vi "UART Read Write.vi"() -> ()   [LabVIEW 2016]
panel:
  in  "Abort":bool
  in  "Start":bool
  out "error out":errorcluster
  in  "Send":bool
  in  "Command":string
  out "concatenated string":string
  in  "stop":bool
  in  "Boolean":bool
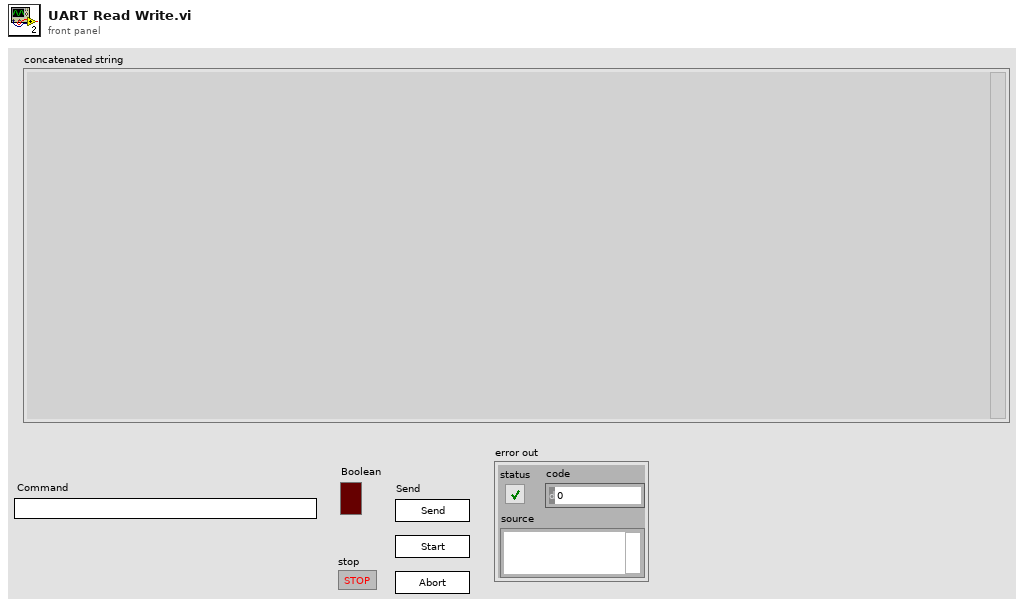
[diagram p1: front panel]
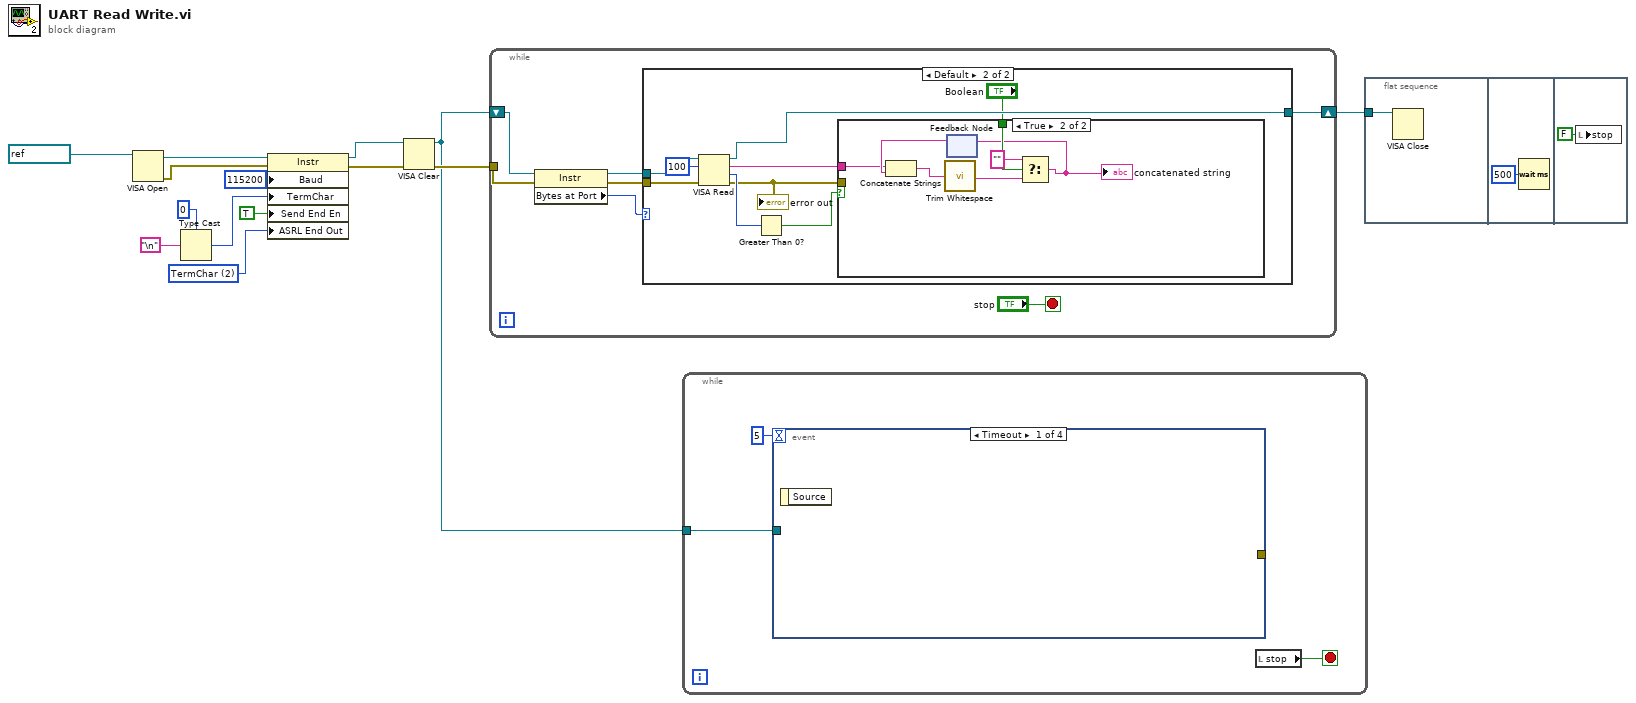
[diagram p0: block diagram]
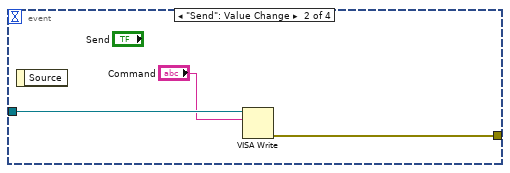
[diagram p2: hidden frame]
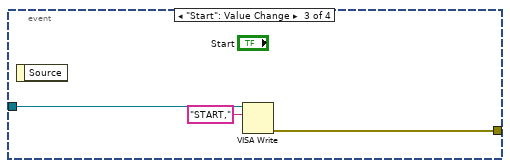
[diagram p3: hidden frame]
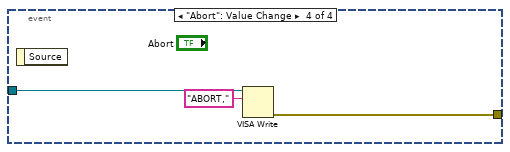
[diagram p4: hidden frame]
diagram:
  w4 = u16 2 items=["None", "Last Bit", "TermChar", "Break"] ("Serial Settings:End Mode for Writes")
  n1 = VISA Open(VISA resource name=refnum<visa-resource-name> "COM3") -> (VISA resource name=w13:refnum<visa-resource-name>, error out=w10:errorcluster)  [unwired: 4 in]
  n2 = Type Cast(type=u8 0 ("Message Based Settings:Termination Character"), x="\n") -> (*(type *) &x=w7:u8)
  n3 = property class="Instr"(reference=w13, error in=w10, "Baud"=u32 115200 ("Serial Settings:Baud Rate"), "TermChar"=w7, "Send End En"=TRUE ("Message Based Settings:Send End Enable"), "ASRL End Out"=w4) -> (reference out=w2:refnum<visa-resource-name>, error out=w11:errorcluster)
  n4 = VISA Clear(VISA resource name=w2, error in (no error)=w11) -> (VISA resource name out=w1:refnum<visa-resource-name>, error out=w3:errorcluster)
  n5 = while {
    tunnel: w3 -> [w17]
    shift-right: [w20] -> w9
    shift-left: w1 -> [w21]
    stop <- "stop" stop-if-true
    n6 = property class="Instr"(reference=w21, error in=w17) -> (reference out=w18:refnum<visa-resource-name>, error out=w16:errorcluster, "Bytes at Port"=w15:u32)
    n7 = case shown="Default" w15 {
      tunnel: [w22 w31] -> w20
      tunnel: w18 -> [w22 w24]
      tunnel: w16 -> [_ w23]
      frame 0 {
      }
      frame Default {
        n8 = VISA Read(VISA resource name=w24, byte count=u32 100, error in (no error)=w23) -> (VISA resource name out=w31:refnum<visa-resource-name>, read buffer=w30:string, return count=w26:u32, error out=w25:errorcluster)
        "error out" <- w25
        n9 = Greater Than 0?(x=w26) -> (x > 0?=w27:bool)
        n10 = case shown="True" w27 {
          tunnel: w30 -> [_ w36]
          tunnel: "Boolean" -> [_ w35]
          tunnel: w25 -> [_ _]
          frame False {
          }
          frame True {
            n11 = feedback #1() -> (w37:string)  [unwired: 1 in]
            n12 = Concatenate Strings(w36, w37) -> (w38:string)
            n13 = call <vilib>:"Trim Whitespace.vi"("string"=w38) -> ("trimmed string"=w34:string)  [unwired: 1 in]
            n14 = Select(t="", s=w35, f=w34) -> (s? t:f=w32:string)
            "concatenated string" <- w32
            n15 = feedback-in #1(w32) -> ()
          }
        }
      }
    }
  }
  n16 = while {
    tunnel: w1 -> [w39]
    stop <- w41 stop-if-true
    n17 = event shown="[0] Timeout" {
      selector: _ -> [_ _ _ _]
      dyn-events: _ -> [_ _ _ _]
      timeout: 5 -> [_ _ _ _]
      tunnel: w39 -> [_ w44 w47 w50]
      tunnel: [_ w42 w46 w49] -> _
      event Timeout {
        n18 = event-data() -> ()  [unwired: 1 in, 1 out]
      }
      event "Send": Value Change {
        n19 = event-data() -> ()  [unwired: 1 in, 1 out]
        n20 = VISA Write(VISA resource name=w44, write buffer="Command") -> (error out=w42:errorcluster)  [unwired: 1 in, 2 out]
      }
      event "Start": Value Change {
        n21 = event-data() -> ()  [unwired: 1 in, 1 out]
        n22 = VISA Write(VISA resource name=w47, write buffer="START,") -> (error out=w46:errorcluster)  [unwired: 1 in, 2 out]
      }
      event "Abort": Value Change {
        n23 = event-data() -> ()  [unwired: 1 in, 1 out]
        n24 = VISA Write(VISA resource name=w50, write buffer="ABORT,") -> (error out=w49:errorcluster)  [unwired: 1 in, 2 out]
      }
    }
    n25 = local read "stop"() -> (w41:bool)
  }
  n26 = flat-sequence {
    tunnel: w9 -> [w51]
    frame #0 {
      n27 = VISA Close(VISA resource name=w51) -> ()  [unwired: 1 in, 1 out]
    }
    frame #1 {
      n28 = Wait (ms)(milliseconds to wait=u32 500) -> ()  [unwired: 1 out]
    }
    frame #2 {
      n29 = local write "stop"(FALSE ("stop")) -> ()
    }
  }
